vi "demo - 副本.vi"() -> ()   [LabVIEW 2019]
uses:
  C:/Users/huang/Desktop/MIL LITE 10/64/Matrox Imaging/MIL/MIL.NET/Matrox.MatroxImagingLibrary.v3.5.dll
  64/Matrox Imaging/MIL/MIL.NET/Matrox.MatroxImagingLibrary.v3.5.dll
panel:
  in  "停止":bool
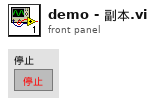
[diagram p1: front panel]
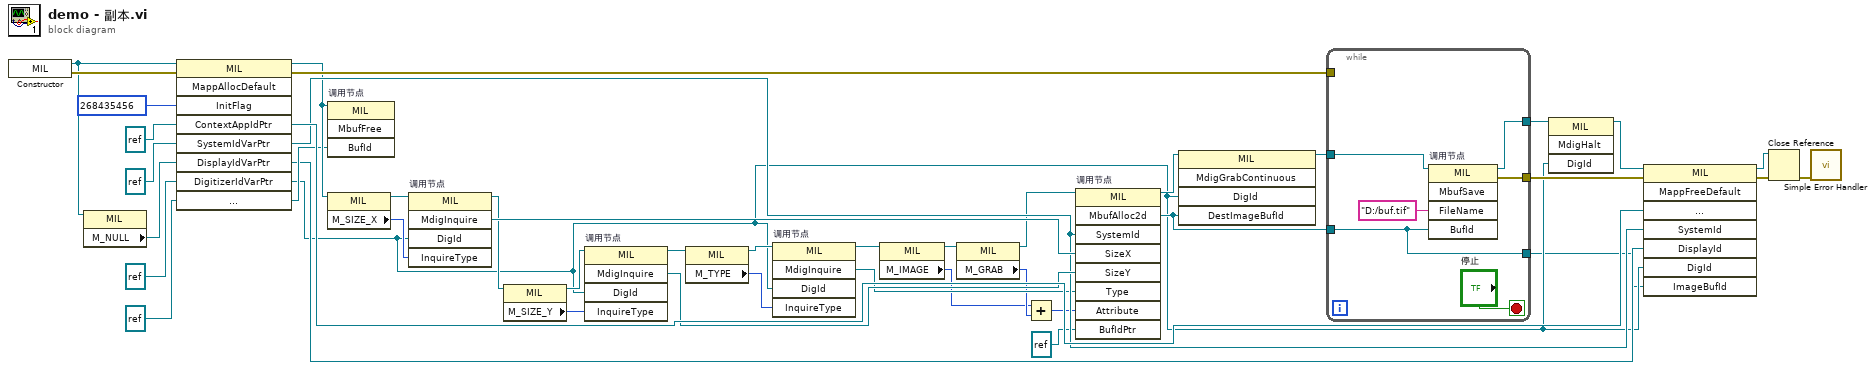
[diagram p0: block diagram]
diagram:
  n1 = constructor class="MIL"() -> (reference out=w12:refnum<k24>, error out=w32:errorcluster)  [unwired: 3 in, 1 out]
  n2 = property class="MIL"(reference=w12) -> ("M_NULL"=w11:refnum<k24>)  [unwired: 1 in, 2 out]
  n3 = invoke on="调用节点" class="MIL" method="MappAllocDefault"(reference=w12, error in=w32, "InitFlag"=i64 268435456, "ContextAppIdPtr"=refnum<k24> refnum, "SystemIdVarPtr"=refnum<k24> refnum, "DisplayIdVarPtr"=w11, "DigitizerIdVarPtr"=refnum<k24> refnum, "ImageIdVarPtr"=refnum<k24> refnum) -> (reference out=w10:refnum<k24>, error out=w36:errorcluster, "ContextAppIdPtr"=w39:refnum<k24>, "SystemIdVarPtr"=w27:refnum<k24>, "DisplayIdVarPtr"=w3:refnum<k24>, "DigitizerIdVarPtr"=w2:refnum<k24>, "ImageIdVarPtr"=w9:refnum<k24>)  [unwired: 1 in, 2 out]
  n4 = invoke on="调用节点" class="MIL" method="MbufFree"(reference=w10, "BufId"=w9) -> ()  [unwired: 2 in, 4 out]
  n5 = property class="MIL"(reference=w10) -> (reference out=w25:refnum<k24>, "M_SIZE_X"=w31:i32)  [unwired: 1 in, 1 out]
  n6 = invoke on="调用节点" class="MIL" method="MdigInquire"(reference=w25, "DigId"=w2, "InquireType"=w31) -> (reference out=w16:refnum<k24>, "MdigInquire"=w29:refnum<k24>)  [unwired: 2 in, 3 out]
  n7 = property class="MIL"(reference=w16) -> (reference out=w26:refnum<k24>, "M_SIZE_Y"=w30:i32)  [unwired: 1 in, 1 out]
  n8 = invoke on="调用节点" class="MIL" method="MdigInquire"(reference=w26, "DigId"=w2, "InquireType"=w30) -> (reference out=w15:refnum<k24>, "MdigInquire"=w28:refnum<k24>)  [unwired: 2 in, 3 out]
  n9 = property class="MIL"(reference=w15) -> (reference out=w24:refnum<k24>, "M_TYPE"=w23:i32)  [unwired: 1 in, 1 out]
  n10 = invoke on="调用节点" class="MIL" method="MdigInquire"(reference=w24, "DigId"=w2, "InquireType"=w23) -> (reference out=w14:refnum<k24>, "MdigInquire"=w22:refnum<k24>)  [unwired: 2 in, 3 out]
  n11 = property class="MIL"(reference=w14) -> (reference out=w17:refnum<k24>, "M_IMAGE"=w19:i32)  [unwired: 1 in, 1 out]
  n12 = property class="MIL"(reference=w17) -> (reference out=w13:refnum<k24>, "M_GRAB"=w20:i32)  [unwired: 1 in, 1 out]
  n13 = Add(x=w19, y=w20) -> (x+y=w18:i32)
  n14 = invoke on="调用节点" class="MIL" method="MbufAlloc2d"(reference=w13, "SystemId"=w27, "SizeX"=w29, "SizeY"=w28, "Type"=w22, "Attribute"=w18, "BufIdPtr"=refnum<k24> refnum) -> (reference out=w8:refnum<k24>, "MbufAlloc2d"=w6:refnum<k24>)  [unwired: 2 in, 7 out]
  n15 = invoke on="调用节点" class="MIL" method="MdigGrabContinuous"(reference=w8, "DigId"=w2, "DestImageBufId"=w6) -> (reference out=w7:refnum<k24>)  [unwired: 2 in, 4 out]
  n16 = while {
    tunnel: [w48] -> w5
    tunnel: w36 -> [_]
    tunnel: [w47] -> w35
    tunnel: w6 -> [w44]
    tunnel: w7 -> [w46]
    tunnel: [w44] -> w1
    stop <- "停止" stop-if-true
    n17 = invoke on="调用节点" class="MIL" method="MbufSave"(reference=w46, "FileName"="D:/buf.tif", "BufId"=w44) -> (reference out=w48:refnum<k24>, error out=w47:errorcluster)  [unwired: 2 in, 3 out]
  }
  n18 = invoke on="调用节点" class="MIL" method="MdigHalt"(reference=w5, "DigId"=w2) -> (reference out=w4:refnum<k24>)  [unwired: 2 in, 3 out]
  n19 = invoke on="调用节点" class="MIL" method="MappFreeDefault"(reference=w4, error in=w35, "ApplicationId"=w39, "SystemId"=w27, "DisplayId"=w3, "DigId"=w2, "ImageBufId"=w1) -> (reference out=w37:refnum<k24>, error out=w34:errorcluster)  [unwired: 1 in, 6 out]
  n20 = Close Reference(reference=w37, error in (no error)=w34) -> (error out=w33:errorcluster)
  n21 = call <vilib>:"Simple Error Handler.vi"("error in (no error)"=w33) -> ()  [unwired: 4 in, 5 out]
